vi "Get Application Build Version.vi"(8 "Error In":errorcluster, 10 "Build Specification Name":string="Application" caption="Build Specification Name (\"Application\")", 11 "Project Filename":string caption="Project Name (Filename Only with Extension)") -> (0 "error out":errorcluster, 2 "Version Numbers":T1, 3 "Version String":string)   [LabVIEW 2016]
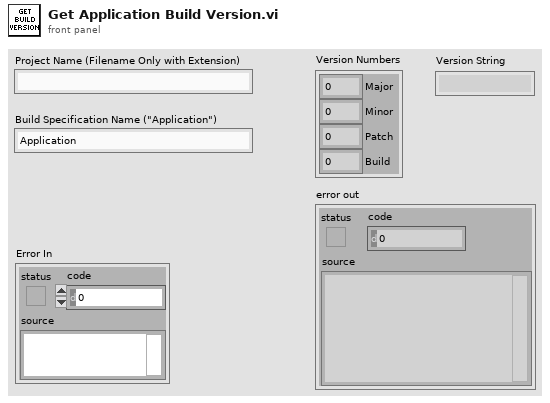
[diagram p1: front panel]
types:
  T1 = cluster{"Major":i32, "Minor":i32, "Patch":i32, "Build":i32}
  T2 = enum32{"invalid app kind", "Development System", "Run Time System", "Student Edition", "Embedded LabVIEW", "Evaluation", "Custom"}
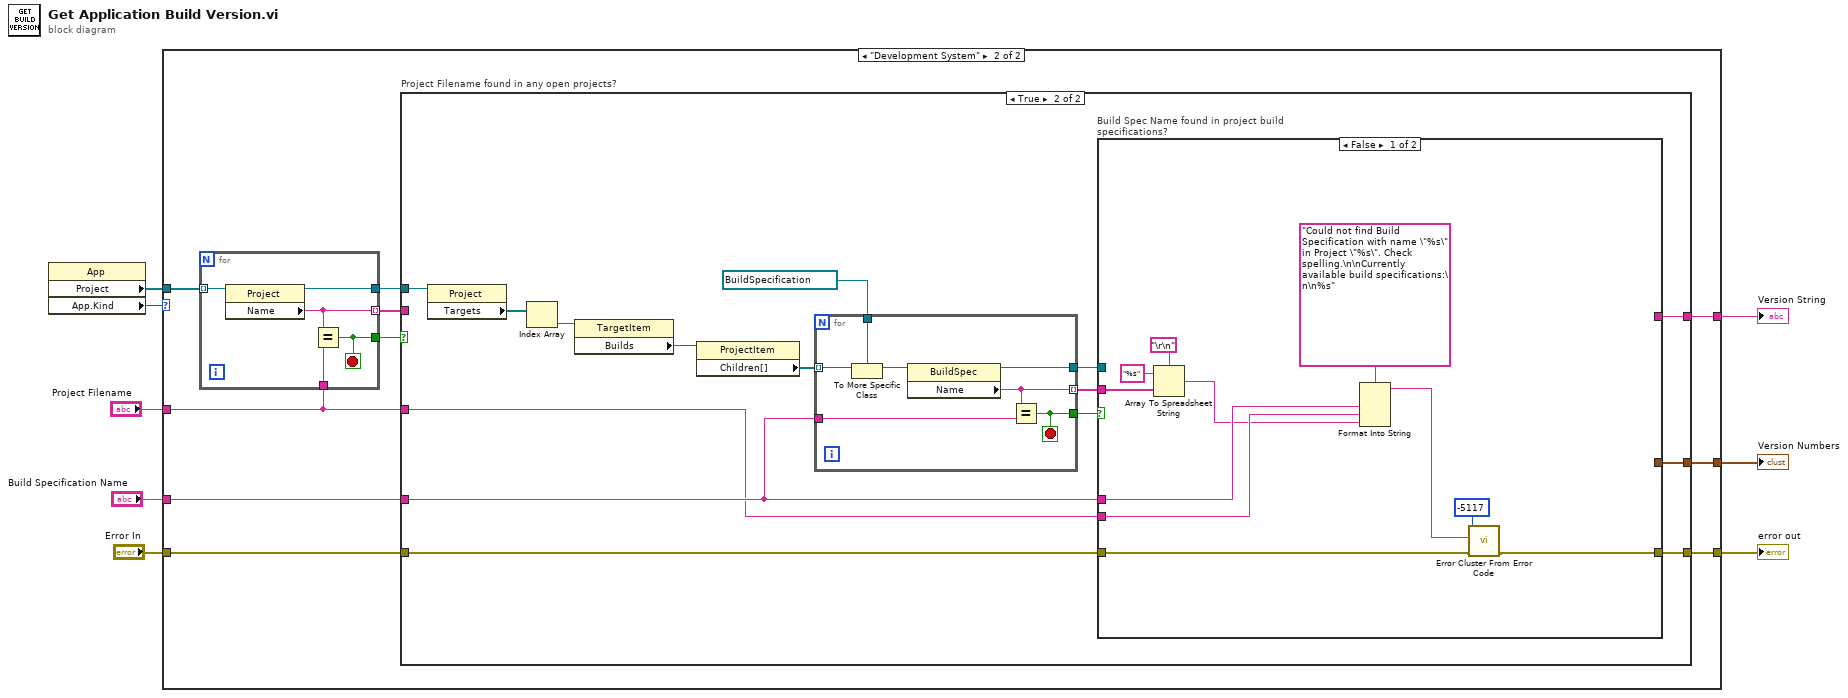
[diagram p0: block diagram]
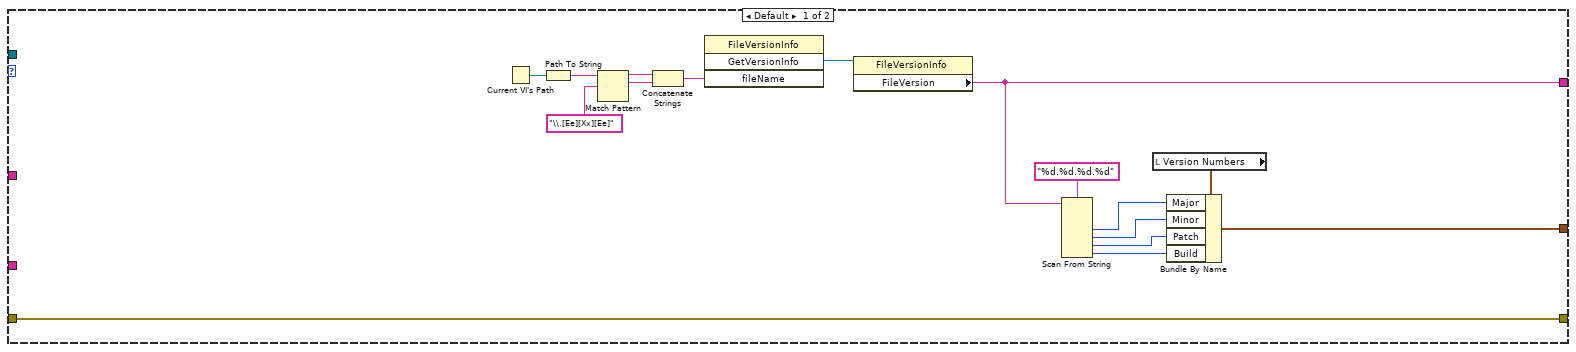
[diagram p2: hidden frame]
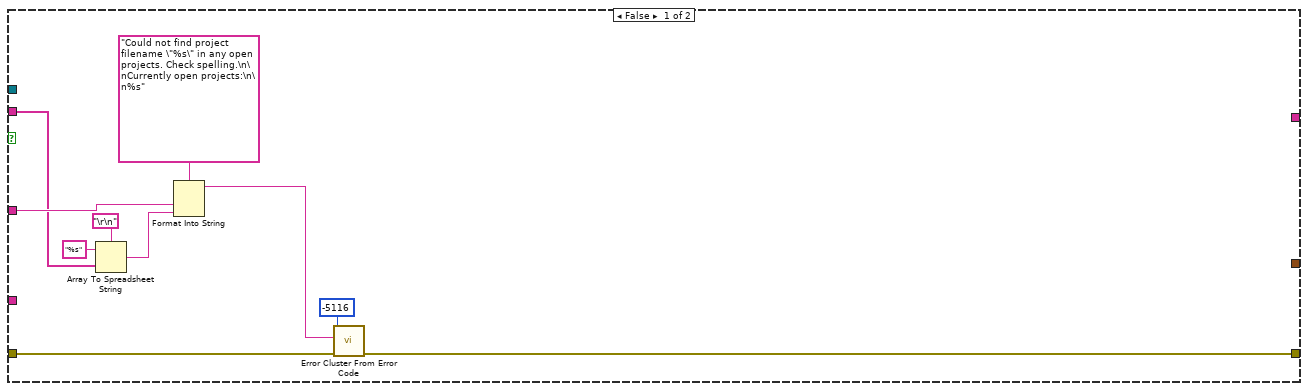
[diagram p3: hidden frame]
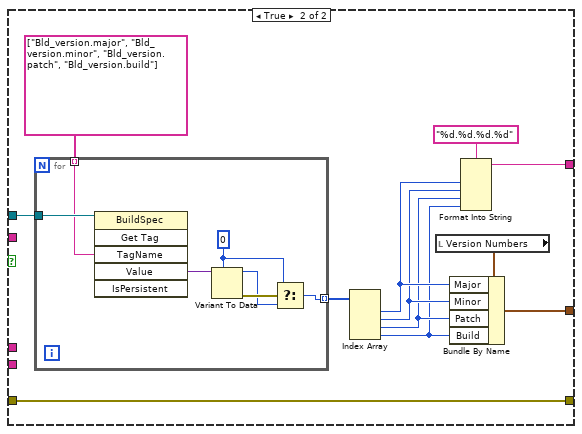
[diagram p4: hidden frame]
diagram:
  n1 = property class="App"() -> ("Project"=w6:refnum<vi>[], "App.Kind"=w1:T2)  [unwired: 2 in, 2 out]
  n2 = case shown="\"Development System\"" w1 {
    tunnel: [w16 w34] -> w8
    tunnel: [w22 w33] -> w7
    tunnel: w6 -> [_ w32]
    tunnel: "Error In" -> [w15 w30]
    tunnel: "Build Specification Name" -> [_ w28]
    tunnel: "Project Filename" -> [_ w27]
    tunnel: [w15 w25] -> w2
    frame Default {
      n3 = Current VI's Path() -> (path=w14:path)
      n4 = Path To String(path=w14) -> (string=w9:string)
      n5 = Match Pattern(string=w9, regular expression="\\.[Ee][Xx][Ee]") -> (before substring=w11:string, match substring=w12:string)  [unwired: 1 in, 2 out]
      n6 = Concatenate Strings(w11, w12) -> (w10:string)
      n7 = invoke class="FileVersionInfo" method="GetVersionInfo"("fileName"=w10) -> ("GetVersionInfo"=w24:refnum<k24>)  [unwired: 3 in, 3 out]
      n8 = property class="FileVersionInfo"(reference=w24) -> ("FileVersion"=w22:string)  [unwired: 1 in, 2 out]
      n9 = Scan From String(format string="%d.%d.%d.%d", input string=w22) -> (output 1=w17:i32, output 2=w18:i32, output 3=w19:i32, output 4=w20:i32)  [unwired: 6 in, 3 out]
      n10 = local read "Version Numbers"() -> (w21:T1)
      n11 = Bundle By Name(cluster=w21, "Major"=w17, "Minor"=w18, "Patch"=w19, "Build"=w20) -> (w16:T1)
    }
    frame "Development System" {
      n12 = for {
        tunnel: w32 -> [w101] mode=indexing
        tunnel: w27 -> [w100]
        tunnel: [w99] -> w31
        tunnel: [w98] -> w29
        tunnel: [w97] -> w26 mode=indexing
        stop <- w99 stop-if-true
        n13 = property class="Project"(reference=w101) -> (reference out=w98:refnum<vi>, "Name"=w97:string)  [unwired: 1 in, 1 out]
        n14 = Equal?(x=w97, y=w100) -> (x = y?=w99:bool)
      }
      n15 = case "Project Filename found in any open projects?" shown="True" w31 {
        tunnel: [_ w52] -> w34
        tunnel: [_ w51] -> w33
        tunnel: [w39 w50] -> w25
        tunnel: w30 -> [w44 w49]
        tunnel: w29 -> [_ w48]
        tunnel: w28 -> [_ w47]
        tunnel: w27 -> [w42 w46]
        tunnel: w26 -> [w38 _]
        frame False {
          n16 = Array To Spreadsheet String(delimiter (Tab)="\r\n", array=w38, 3:"%s" ("format string")) -> (spreadsheet string=w36:string)
          n17 = Format Into String(format string="Could not find project filename \"%s\" in any open projects. Check spelling.\n\nCurrently open projects:\n\n%s", w42, w36) -> (resulting string=w40:string)  [unwired: 2 in, 1 out]
          n18 = call <vilib>:"Error Cluster From Error Code.vi"("error in (no error)"=w44, "error message (\"\")"=w40, "error code (0)"=-5116 ("error code (-5001)")) -> ("error out"=w39:errorcluster)  [unwired: 6 in]
        }
        frame True {
          n19 = property class="Project"(reference=w48) -> ("Targets"=w59:refnum<vi>[])  [unwired: 1 in, 2 out]
          n20 = Index Array(array=w59) -> (element=w58:refnum<vi>)  [unwired: 1 in]
          n21 = property class="TargetItem"(reference=w58) -> ("Builds"=w57:refnum<vi>)  [unwired: 1 in, 2 out]
          n22 = property class="ProjectItem"(reference=w57) -> ("Children[]"=w56:refnum<vi>[])  [unwired: 1 in, 2 out]
          n23 = for {
            tunnel: w56 -> [w96] mode=indexing
            tunnel: refnum<vi> refnum ("reference") -> [w94]
            tunnel: [w93] -> w54
            tunnel: [w92] -> w53
            tunnel: w47 -> [w91]
            tunnel: [w90] -> w45 mode=indexing
            stop <- w92 stop-if-true
            n24 = To More Specific Class(target class=w94, reference=w96) -> (specific class reference=w95:refnum<vi>)  [unwired: 1 in, 1 out]
            n25 = property class="BuildSpec"(reference=w95) -> (reference out=w93:refnum<vi>, "Name"=w90:string)  [unwired: 1 in, 1 out]
            n26 = Equal?(x=w90, y=w91) -> (x = y?=w92:bool)
          }
          n27 = case "Build Spec Name found in project build specifications?" shown="False" w53 {
            tunnel: w54 -> [_ w82]
            tunnel: [_ w78] -> w52
            tunnel: [_ w72] -> w51
            tunnel: [w62 w71] -> w50
            tunnel: w49 -> [w61 w71]
            tunnel: w47 -> [w69 _]
            tunnel: w46 -> [w68 _]
            tunnel: w45 -> [w65 _]
            frame False {
              n28 = Array To Spreadsheet String(delimiter (Tab)="\r\n", array=w65, 3:"%s" ("format string")) -> (spreadsheet string=w64:string)
              n29 = Format Into String(format string="Could not find Build Specification with name \"%s\" in Project \"%s\". Check spelling.\n\nCurrently available build specifications:\n\n%s", w69, w68, w64) -> (resulting string=w60:string)  [unwired: 2 in, 1 out]
              n30 = call <vilib>:"Error Cluster From Error Code.vi"("error in (no error)"=w61, "error message (\"\")"=w60, "error code (0)"=-5117 ("error code (-5001)")) -> ("error out"=w62:errorcluster)  [unwired: 6 in]
            }
            frame True {
              n31 = for {
                tunnel: w82 -> [w89]
                tunnel: string[] ["Bld_version.major", "Bld_version.minor", "Bld_version.patch", "Bld_version.build"] -> [w88] mode=indexing
                tunnel: [w83] -> w80 mode=indexing
                w85 = 0
                n32 = invoke class="BuildSpec" method="Get Tag"(reference=w89, "TagName"=w88) -> ("Value"=w87:variant)  [unwired: 4 in, 5 out]
                n33 = Variant To Data(type=w85, Variant=w87) -> (data=w84:i32, error out=w86:errorcluster)  [unwired: 1 in]
                n34 = Select(t=w85, s=w86, f=w84) -> (s? t:f=w83:i32)
              }
              n35 = Index Array(array=w80) -> (element #1=w76:i32, element #2=w75:i32, element #3=w74:i32, element #4=w73:i32)  [unwired: 4 in]
              n36 = local read "Version Numbers"() -> (w79:T1)
              n37 = Bundle By Name(cluster=w79, "Major"=w76, "Minor"=w75, "Patch"=w74, "Build"=w73) -> (w78:T1)
              n38 = Format Into String(format string="%d.%d.%d.%d", w76, w75, w74, w73) -> (resulting string=w72:string)  [unwired: 2 in, 1 out]
            }
          }
        }
      }
    }
  }
  "Version String" <- w7
  "Version Numbers" <- w8
  "error out" <- w2
